vi "Create New Record.Error.vi"(6 "Display Format":T1, 7 "Record.Error in":refnum<class "Record.Error.lvclass">, 8 "error in (no error)":errorcluster, 9 "Error":errorcluster, 10 "Message":string, 11 "Level":T2(ring)) -> (0 "error out":errorcluster, 3 "Record.Error out":refnum<class "Record.Error.lvclass">)   [LabVIEW 2017, in "Error Log.lvlib" / "Record.Error.lvclass"]
uses:
  Record.Error.lvclass
  Serializer/Type Defs/Display Format.ctl
  Serializer/Serializer.lvclass
  Serializer/Serializer.lvlib
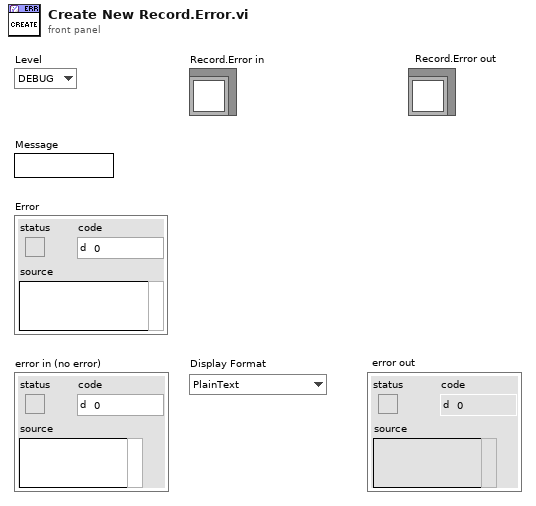
[diagram p1: front panel]
types:
  T1 = typedef "Serializer.lvlib/Display Format.ctl" = enum16{"PlainText", "PlainText.INI", "XML", "JSON"}
  T2 = enum16{"DEBUG", "INFO", "WARNING", "ERROR", "CRITICAL"}
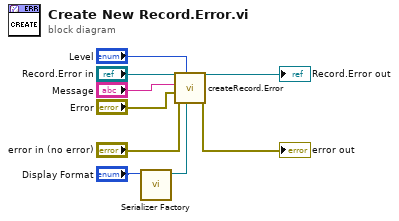
[diagram p0: block diagram]
diagram:
  n1 = call "Serializer Factory.vi"("Display Format"="Display Format") -> ("Serializer"=w1:refnum<class "Serializer.lvclass">)  [unwired: 9 in, 1 out]
  n2 = call-dynamic "createRecord.Error.vi"("Serializer"=w1, "Level"="Level", "error in (no error)"="error in (no error)", "Error"="Error", "Message"="Message", "Record.Error in"="Record.Error in") -> ("error out"=→"error out":errorcluster, "Record.Error out"=→"Record.Error out":refnum<class "Record.Error.lvclass">)  [unwired: 4 in]
